vi "driveTrainControl.vi"(6 "driveTrainKillButton":bool, 7 "ClosedLoopMaxOutput":dbl, 8 "backRight":T1={"DeviceStatus"={"status"=FALSE, "code"=0, "source"=""}, "Type"=enum."PWM", "PWM"={"Digital Module"=enum."Digital Module 2", "PWM Channel"=enum."PWM 1", "DeadBand"={"Name"="", "maxPositivePwm"=0, "minPositivePwm"=0, "centerPwm"=0, "maxNegativePwm"=0, "minNegativePwm"=0, "angularRange"=0}}, "CAN"={"Device Number"=0, "Control Mode"=enum."Percent VBus", "Semaphore"=refnum, "Max Vout"=12.0}, "Invert"=FALSE, "TransformRef"=refnum, "InvTransformRef"=refnum}, 9 "backLeft":T1={"DeviceStatus"={"status"=FALSE, "code"=0, "source"=""}, "Type"=enum."PWM", "PWM"={"Digital Module"=enum."Digital Module 2", "PWM Channel"=enum."PWM 1", "DeadBand"={"Name"="", "maxPositivePwm"=0, "minPositivePwm"=0, "centerPwm"=0, "maxNegativePwm"=0, "minNegativePwm"=0, "angularRange"=0}}, "CAN"={"Device Number"=0, "Control Mode"=enum."Percent VBus", "Semaphore"=refnum, "Max Vout"=12.0}, "Invert"=FALSE, "TransformRef"=refnum, "InvTransformRef"=refnum}, 10 "frontRight":T1={"DeviceStatus"={"status"=FALSE, "code"=0, "source"=""}, "Type"=enum."PWM", "PWM"={"Digital Module"=enum."Digital Module 2", "PWM Channel"=enum."PWM 1", "DeadBand"={"Name"="", "maxPositivePwm"=0, "minPositivePwm"=0, "centerPwm"=0, "maxNegativePwm"=0, "minNegativePwm"=0, "angularRange"=0}}, "CAN"={"Device Number"=0, "Control Mode"=enum."Percent VBus", "Semaphore"=refnum, "Max Vout"=12.0}, "Invert"=FALSE, "TransformRef"=refnum, "InvTransformRef"=refnum}, 11 "frontLeft":T1={"DeviceStatus"={"status"=FALSE, "code"=0, "source"=""}, "Type"=enum."PWM", "PWM"={"Digital Module"=enum."Digital Module 2", "PWM Channel"=enum."PWM 1", "DeadBand"={"Name"="", "maxPositivePwm"=0, "minPositivePwm"=0, "centerPwm"=0, "maxNegativePwm"=0, "minNegativePwm"=0, "angularRange"=0}}, "CAN"={"Device Number"=0, "Control Mode"=enum."Percent VBus", "Semaphore"=refnum, "Max Vout"=12.0}, "Invert"=FALSE, "TransformRef"=refnum, "InvTransformRef"=refnum}) -> (0 "backRight":T1={"DeviceStatus"={"status"=FALSE, "code"=0, "source"=""}, "Type"=enum."PWM", "PWM"={"Digital Module"=enum."Digital Module 1", "PWM Channel"=enum."Invalid", "DeadBand"={"Name"="", "maxPositivePwm"=0, "minPositivePwm"=0, "centerPwm"=0, "maxNegativePwm"=0, "minNegativePwm"=0, "angularRange"=0}}, "CAN"={"Device Number"=0, "Control Mode"=enum."Percent VBus", "Semaphore"=refnum, "Max Vout"=12.0}, "Invert"=FALSE, "TransformRef"=refnum, "InvTransformRef"=refnum}, 1 "backLeft":T1={"DeviceStatus"={"status"=FALSE, "code"=0, "source"=""}, "Type"=enum."PWM", "PWM"={"Digital Module"=enum."Digital Module 1", "PWM Channel"=enum."Invalid", "DeadBand"={"Name"="", "maxPositivePwm"=0, "minPositivePwm"=0, "centerPwm"=0, "maxNegativePwm"=0, "minNegativePwm"=0, "angularRange"=0}}, "CAN"={"Device Number"=0, "Control Mode"=enum."Percent VBus", "Semaphore"=refnum, "Max Vout"=12.0}, "Invert"=FALSE, "TransformRef"=refnum, "InvTransformRef"=refnum}, 2 "frontRight":T1={"DeviceStatus"={"status"=FALSE, "code"=0, "source"=""}, "Type"=enum."PWM", "PWM"={"Digital Module"=enum."Digital Module 1", "PWM Channel"=enum."Invalid", "DeadBand"={"Name"="", "maxPositivePwm"=0, "minPositivePwm"=0, "centerPwm"=0, "maxNegativePwm"=0, "minNegativePwm"=0, "angularRange"=0}}, "CAN"={"Device Number"=0, "Control Mode"=enum."Percent VBus", "Semaphore"=refnum, "Max Vout"=12.0}, "Invert"=FALSE, "TransformRef"=refnum, "InvTransformRef"=refnum}, 3 "frontLeft":T1={"DeviceStatus"={"status"=FALSE, "code"=0, "source"=""}, "Type"=enum."PWM", "PWM"={"Digital Module"=enum."Digital Module 1", "PWM Channel"=enum."Invalid", "DeadBand"={"Name"="", "maxPositivePwm"=0, "minPositivePwm"=0, "centerPwm"=0, "maxNegativePwm"=0, "minNegativePwm"=0, "angularRange"=0}}, "CAN"={"Device Number"=0, "Control Mode"=enum."Percent VBus", "Semaphore"=refnum, "Max Vout"=12.0}, "Invert"=FALSE, "TransformRef"=refnum, "InvTransformRef"=refnum}, 5 "drivetrainMaxOutput":dbl)   [LabVIEW 2012]
uses:
  <vilib>/Rock Robotics/WPI/MotorControl/WPI_MotorControlDeviceRef.ctl
  <vilib>/Rock Robotics/SystemInterfaces/Typedef/FPGA_TypedefDigitalModule.ctl
  <vilib>/Rock Robotics/SystemInterfaces/DIO/FPGA_DIOPWMChannel.ctl
  <vilib>/Rock Robotics/WPI/PWM/WPI_PWMDeadband.ctl
  <vilib>/Rock Robotics/WPI/CAN/Jaguar/SubVIs/WPI_CANJaguar_ControlMode.ctl
  <vilib>/Rock Robotics/WPI/PWM/WPI_PWMTransform_ConPane.ctl
  <vilib>/Rock Robotics/WPI/CAN/Jaguar/SubVIs/WPI_CANJaguar_SpeedReference.ctl
  2013NewCan/Robot Global Data.vi
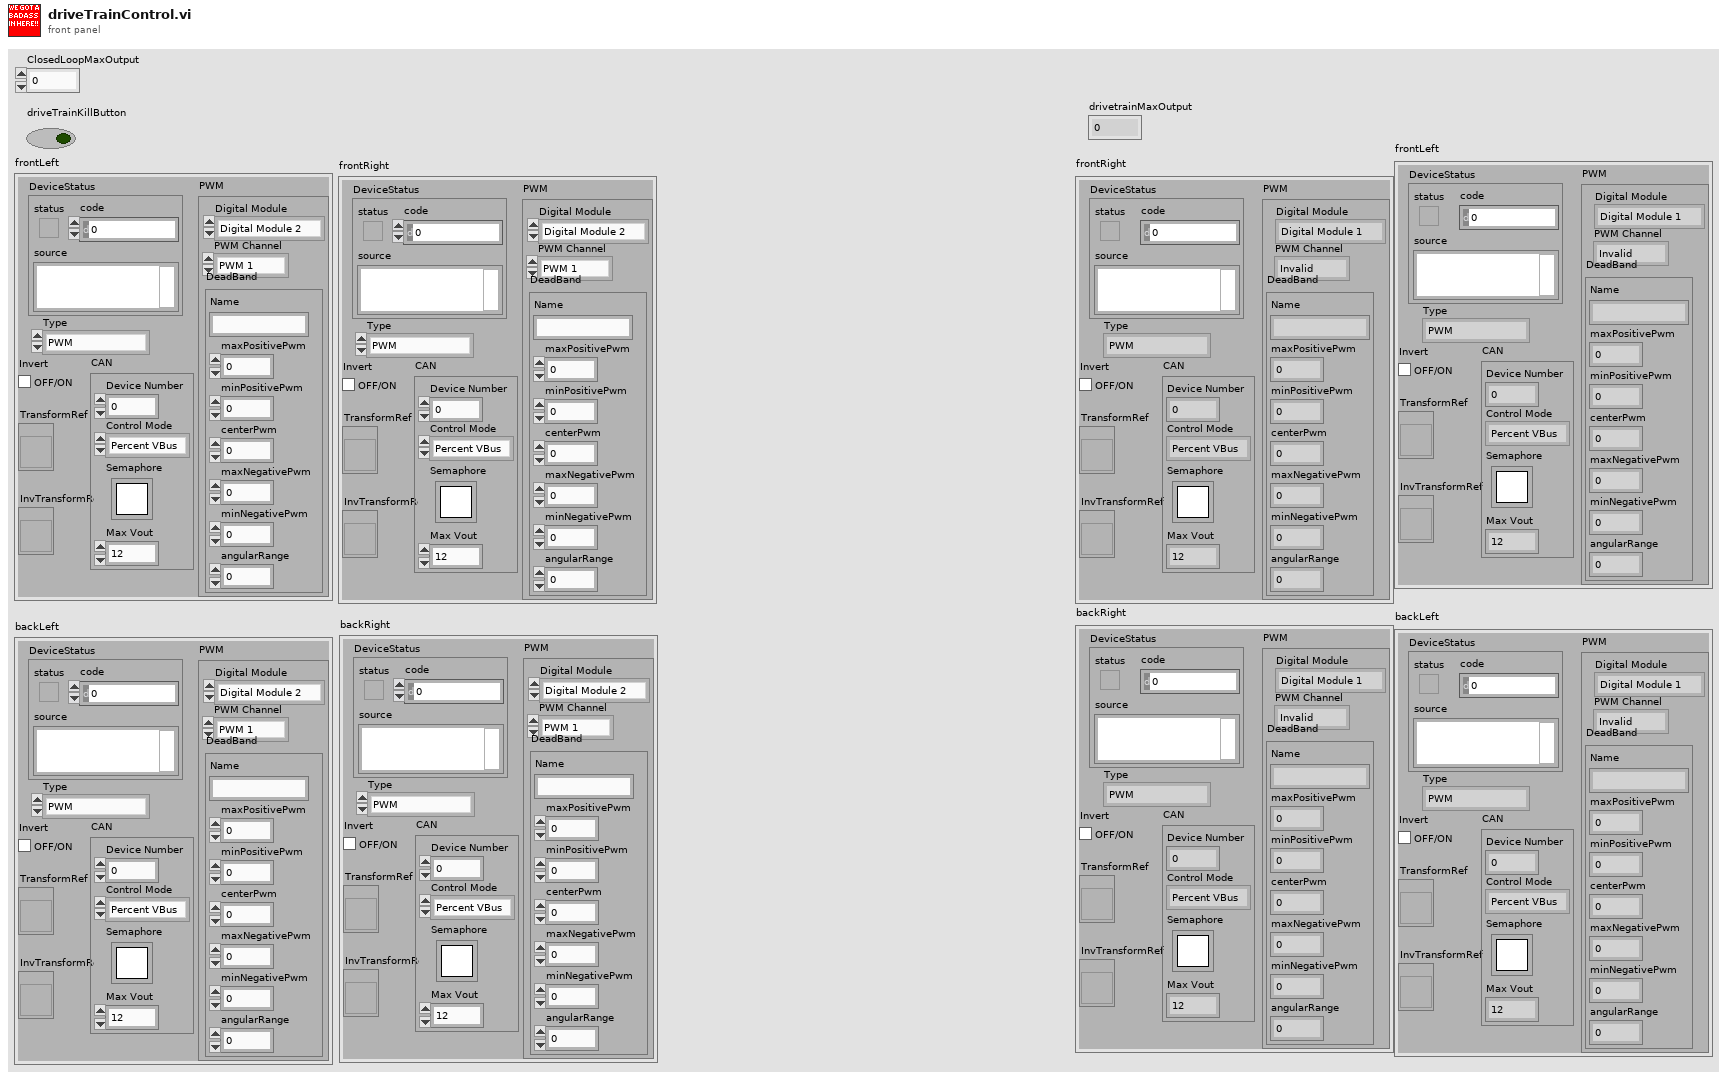
[diagram p1: front panel]
types:
  T1 = typedef "WPI_MotorControlDeviceRef.ctl" = cluster{"DeviceStatus":errorcluster, "Type":enum16{"PWM", "CAN"}, "PWM":cluster{"Digital Module":T2, "PWM Channel":T3, "DeadBand":T4}, "CAN":cluster{"Device Number":u8, "Control Mode":T5, "Semaphore":T6, "Max Vout":dbl}, "Invert":bool, "TransformRef":T7, "InvTransformRef":T7}
  T2 = typedef "FPGA_TypedefDigitalModule.ctl" = enum16{"Digital Module 1", "Digital Module 2"}
  T3 = typedef "FPGA_DIOPWMChannel.ctl" = enum8{"PWM 1", "PWM 2", "PWM 3", "PWM 4", "PWM 5", "PWM 6", "PWM 7", "PWM 8", "PWM 9", "PWM 10", "Invalid"}
  T4 = typedef "WPI_PWMDeadband.ctl" = cluster{"Name":string, "maxPositivePwm":i32, "minPositivePwm":i32, "centerPwm":i32, "maxNegativePwm":i32, "minNegativePwm":i32, "angularRange":u16}
  T5 = typedef "WPI_CANJaguar_ControlMode.ctl" = enum8{"Percent VBus", "Current", "Speed", "Position", "Voltage"}
  T6 = typedef "Semaphore RefNum" = refnum<k1>
  T7 = typedef "WPI_PWMTransform_ConPane.ctl" = refnum<vi>
  T8 = typedef "WPI_CANJaguar_SpeedReference.ctl" = u8
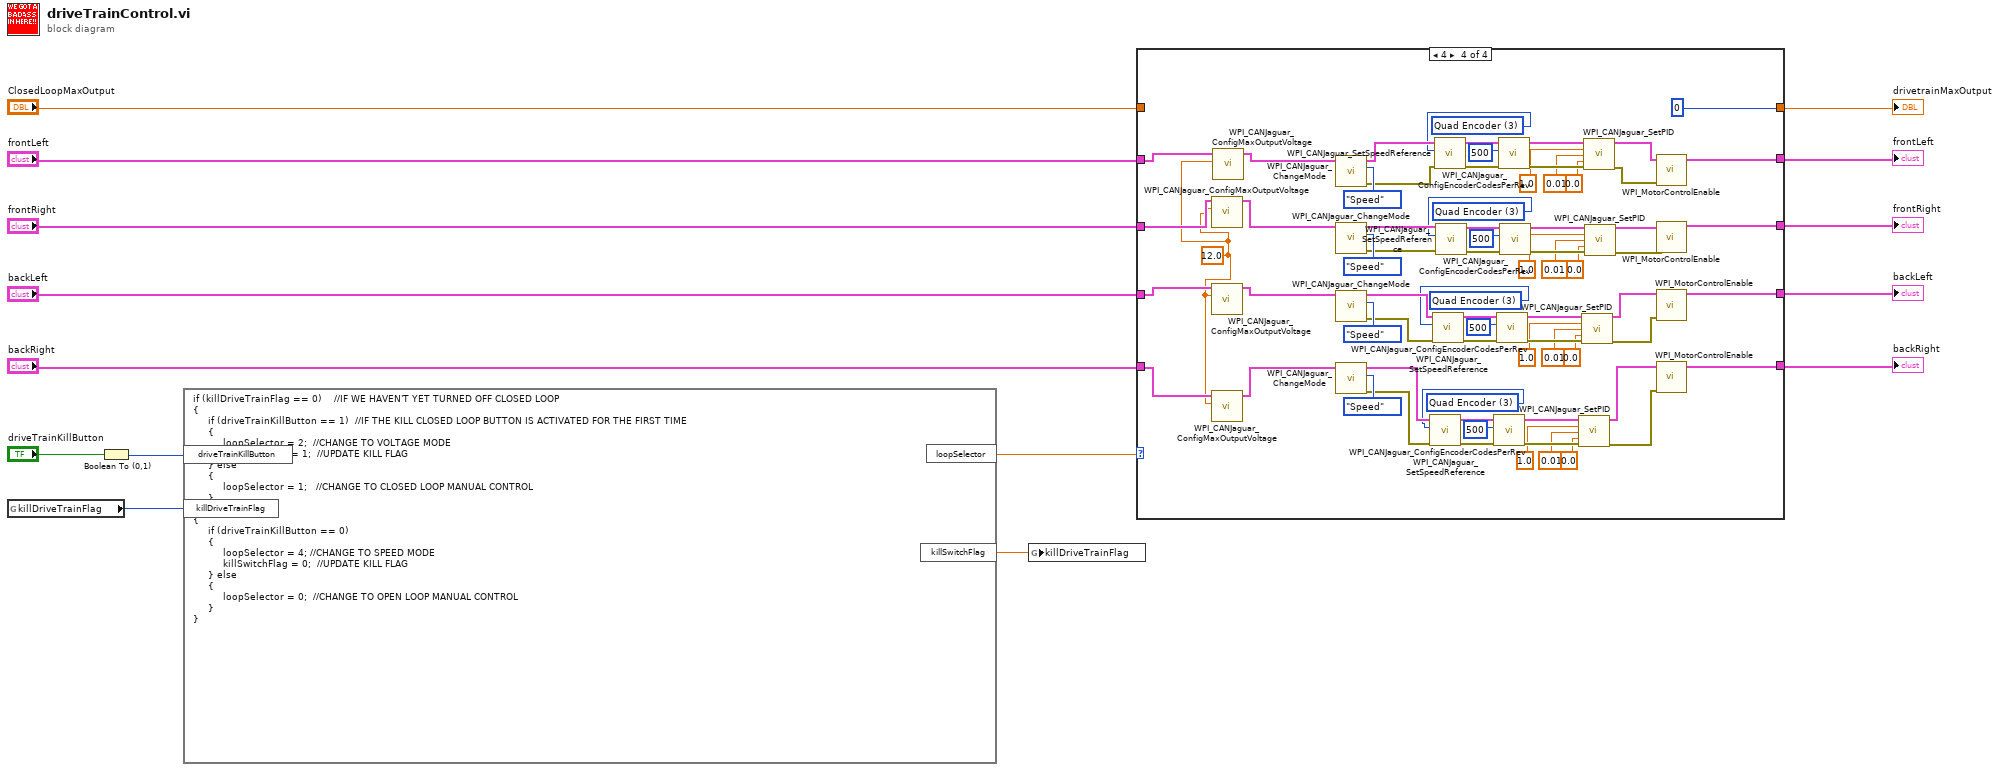
[diagram p0: block diagram]
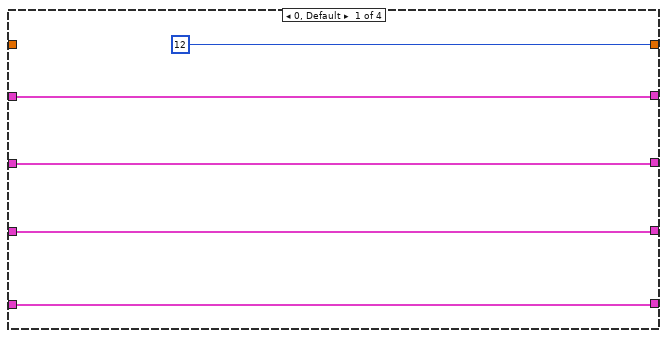
[diagram p2: hidden frame]
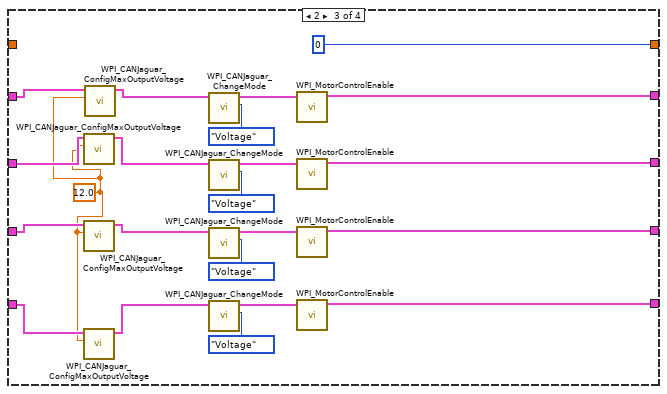
[diagram p4: hidden frame]
diagram:
  n1 = global read "Robot Global Data.vi" "killDriveTrainFlag"() -> (w9:i8)
  n2 = Boolean To (0,1)(Boolean="driveTrainKillButton") -> (0, 1=w11:i16)
  n3 = formula code="if (killDriveTrainFlag == 0)    //IF WE HAVEN'T YET TURNED OFF CLOSED LOOP\n{\n     if (driveTrainKillButton == 1)  //IF THE KILL CLOSED LOOP BUTTON IS ACTIVATED FOR THE FIRST TIME\n     {\n          loopSelector = 2;  //CHANGE TO VOLTAGE MODE\n          killSwitchFlag = 1;  //UPDATE KILL FLAG\n     } else\n     {\n          loopSelector = 1;   //CHANGE TO CLOSED LOOP MANUAL CONTROL\n     }\n} else\n{\n     if (driveTrainKillButton == 0)\n     {\n          loopSelector = 4; //CHANGE TO SPEED MODE\n          killSwitchFlag = 0;  //UPDATE KILL FLAG\n     } else\n     {\n          loopSelector = 0;  //CHANGE TO OPEN LOOP MANUAL CONTROL\n     }\n}"("driveTrainKillButton"=w11, "killDriveTrainFlag"=w9) -> ("loopSelector"=w1:dbl, "killSwitchFlag"=w8:dbl)
  n4 = global write "Robot Global Data.vi" "killDriveTrainFlag"(w8) -> ()
  n5 = case shown="4" w1 {
    tunnel: "frontLeft" -> [w20 w24 w34 w108]
    tunnel: "frontRight" -> [w19 w23 w33 w107]
    tunnel: "backLeft" -> [w18 w22 w32 w106]
    tunnel: "backRight" -> [w17 w21 w31 w105]
    tunnel: [w18 w22 w39 w113] -> w7
    tunnel: [w19 w23 w38 w112] -> w6
    tunnel: [w20 w24 w37 w111] -> w5
    tunnel: [w17 w21 w36 w110] -> w4
    tunnel: [12 w25 0 0] -> w3
    tunnel: "ClosedLoopMaxOutput" -> [_ w25 _ _]
    frame 0, Default {
    }
    frame 1 {
    }
    frame 2 {
      w26 = 12.0 ("Maximum Output Voltage")
      n6 = call <vilib>:"WPI_CANJaguar_ConfigMaxOutputVoltage.vi"("Maximum Output Voltage"=w26, "CAN Jaguar Ref"=w33) -> ("CAN Jaguar Ref Out"=w28:T1)  [unwired: 8 in, 1 out]
      n7 = call <vilib>:"WPI_CANJaguar_ConfigMaxOutputVoltage.vi"("Maximum Output Voltage"=w26, "CAN Jaguar Ref"=w32) -> ("CAN Jaguar Ref Out"=w29:T1)  [unwired: 8 in, 1 out]
      n8 = call <vilib>:"WPI_CANJaguar_ConfigMaxOutputVoltage.vi"("Maximum Output Voltage"=w26, "CAN Jaguar Ref"=w31) -> ("CAN Jaguar Ref Out"=w30:T1)  [unwired: 8 in, 1 out]
      n9 = call <vilib>:"WPI_CANJaguar_ConfigMaxOutputVoltage.vi"("Maximum Output Voltage"=w26, "CAN Jaguar Ref"=w34) -> ("CAN Jaguar Ref Out"=w27:T1)  [unwired: 8 in, 1 out]
      n10 = call <vilib>:"WPI_CANJaguar_ChangeMode.vi"("Control Mode"=WPI_CANJaguar_ControlMode."Voltage", "CAN Jaguar Ref"=w27) -> ("CAN Jaguar Ref Out"=w46:T1)  [unwired: 8 in, 1 out]
      n11 = call <vilib>:"WPI_CANJaguar_ChangeMode.vi"("Control Mode"=WPI_CANJaguar_ControlMode."Voltage", "CAN Jaguar Ref"=w28) -> ("CAN Jaguar Ref Out"=w44:T1)  [unwired: 8 in, 1 out]
      n12 = call <vilib>:"WPI_CANJaguar_ChangeMode.vi"("Control Mode"=WPI_CANJaguar_ControlMode."Voltage", "CAN Jaguar Ref"=w29) -> ("CAN Jaguar Ref Out"=w42:T1)  [unwired: 8 in, 1 out]
      n13 = call <vilib>:"WPI_CANJaguar_ChangeMode.vi"("Control Mode"=WPI_CANJaguar_ControlMode."Voltage", "CAN Jaguar Ref"=w30) -> ("CAN Jaguar Ref Out"=w40:T1)  [unwired: 8 in, 1 out]
      n14 = call <vilib>:"WPI_MotorControlEnable.vi"("CAN Jaguar Ref"=w46) -> ("CAN Jaguar Ref Out"=w37:T1)  [unwired: 9 in, 1 out]
      n15 = call <vilib>:"WPI_MotorControlEnable.vi"("CAN Jaguar Ref"=w44) -> ("CAN Jaguar Ref Out"=w38:T1)  [unwired: 9 in, 1 out]
      n16 = call <vilib>:"WPI_MotorControlEnable.vi"("CAN Jaguar Ref"=w42) -> ("CAN Jaguar Ref Out"=w39:T1)  [unwired: 9 in, 1 out]
      n17 = call <vilib>:"WPI_MotorControlEnable.vi"("CAN Jaguar Ref"=w40) -> ("CAN Jaguar Ref Out"=w36:T1)  [unwired: 9 in, 1 out]
    }
    frame 4 {
      w48 = T8 3 items=["Encoder"=0, "Inv Encoder"=2, "Quad Encoder"=3, "None"=255] ("Speed Reference")
      w49 = T8 3 items=["Encoder"=0, "Inv Encoder"=2, "Quad Encoder"=3, "None"=255] ("Speed Reference")
      w50 = T8 3 items=["Encoder"=0, "Inv Encoder"=2, "Quad Encoder"=3, "None"=255] ("Speed Reference")
      w51 = T8 3 items=["Encoder"=0, "Inv Encoder"=2, "Quad Encoder"=3, "None"=255] ("Speed Reference")
      w100 = 12.0 ("Maximum Output Voltage")
      n18 = call <vilib>:"WPI_CANJaguar_ConfigMaxOutputVoltage.vi"("Maximum Output Voltage"=w100, "CAN Jaguar Ref"=w107) -> ("CAN Jaguar Ref Out"=w102:T1)  [unwired: 8 in, 1 out]
      n19 = call <vilib>:"WPI_CANJaguar_ConfigMaxOutputVoltage.vi"("Maximum Output Voltage"=w100, "CAN Jaguar Ref"=w106) -> ("CAN Jaguar Ref Out"=w103:T1)  [unwired: 8 in, 1 out]
      n20 = call <vilib>:"WPI_CANJaguar_ConfigMaxOutputVoltage.vi"("Maximum Output Voltage"=w100, "CAN Jaguar Ref"=w105) -> ("CAN Jaguar Ref Out"=w104:T1)  [unwired: 8 in, 1 out]
      n21 = call <vilib>:"WPI_CANJaguar_ConfigMaxOutputVoltage.vi"("Maximum Output Voltage"=w100, "CAN Jaguar Ref"=w108) -> ("CAN Jaguar Ref Out"=w101:T1)  [unwired: 8 in, 1 out]
      n22 = call <vilib>:"WPI_CANJaguar_ChangeMode.vi"("Control Mode"=WPI_CANJaguar_ControlMode."Speed", "CAN Jaguar Ref"=w101) -> ("error out"=w65:errorcluster, "CAN Jaguar Ref Out"=w67:T1)  [unwired: 8 in]
      n23 = call <vilib>:"WPI_CANJaguar_ChangeMode.vi"("Control Mode"=WPI_CANJaguar_ControlMode."Speed", "CAN Jaguar Ref"=w102) -> ("error out"=w64:errorcluster, "CAN Jaguar Ref Out"=w66:T1)  [unwired: 8 in]
      n24 = call <vilib>:"WPI_CANJaguar_ChangeMode.vi"("Control Mode"=WPI_CANJaguar_ControlMode."Speed", "CAN Jaguar Ref"=w103) -> ("error out"=w62:errorcluster, "CAN Jaguar Ref Out"=w63:T1)  [unwired: 8 in]
      n25 = call <vilib>:"WPI_CANJaguar_ChangeMode.vi"("Control Mode"=WPI_CANJaguar_ControlMode."Speed", "CAN Jaguar Ref"=w104) -> ("error out"=w60:errorcluster, "CAN Jaguar Ref Out"=w61:T1)  [unwired: 8 in]
      n26 = call <vilib>:"WPI_CANJaguar_SetSpeedReference.vi"("error in (no error)"=w60, "Speed Reference"=w48, "CAN Jaguar Ref"=w61) -> ("error out"=w70:errorcluster, "CAN Jaguar Ref Out"=w69:T1)  [unwired: 7 in]
      n27 = call <vilib>:"WPI_CANJaguar_SetSpeedReference.vi"("error in (no error)"=w62, "Speed Reference"=w49, "CAN Jaguar Ref"=w63) -> ("error out"=w78:errorcluster, "CAN Jaguar Ref Out"=w77:T1)  [unwired: 7 in]
      n28 = call <vilib>:"WPI_CANJaguar_SetSpeedReference.vi"("error in (no error)"=w65, "Speed Reference"=w51, "CAN Jaguar Ref"=w67) -> ("error out"=w94:errorcluster, "CAN Jaguar Ref Out"=w93:T1)  [unwired: 7 in]
      n29 = call <vilib>:"WPI_CANJaguar_SetSpeedReference.vi"("error in (no error)"=w64, "Speed Reference"=w50, "CAN Jaguar Ref"=w66) -> ("error out"=w86:errorcluster, "CAN Jaguar Ref Out"=w85:T1)  [unwired: 7 in]
      n30 = call <vilib>:"WPI_CANJaguar_ConfigEncoderCodesPerRev.vi"("error in (no error)"=w70, "Encoder Codes Per Rev"=u16 500, "CAN Jaguar Ref"=w69) -> ("error out"=w74:errorcluster, "CAN Jaguar Ref Out"=w68:T1)  [unwired: 7 in]
      n31 = call <vilib>:"WPI_CANJaguar_ConfigEncoderCodesPerRev.vi"("error in (no error)"=w78, "Encoder Codes Per Rev"=u16 500, "CAN Jaguar Ref"=w77) -> ("error out"=w82:errorcluster, "CAN Jaguar Ref Out"=w76:T1)  [unwired: 7 in]
      n32 = call <vilib>:"WPI_CANJaguar_ConfigEncoderCodesPerRev.vi"("error in (no error)"=w94, "Encoder Codes Per Rev"=u16 500, "CAN Jaguar Ref"=w93) -> ("error out"=w98:errorcluster, "CAN Jaguar Ref Out"=w92:T1)  [unwired: 7 in]
      n33 = call <vilib>:"WPI_CANJaguar_ConfigEncoderCodesPerRev.vi"("error in (no error)"=w86, "Encoder Codes Per Rev"=u16 500, "CAN Jaguar Ref"=w85) -> ("error out"=w90:errorcluster, "CAN Jaguar Ref Out"=w84:T1)  [unwired: 7 in]
      n34 = call <vilib>:"WPI_CANJaguar_SetPID.vi"("CAN Jaguar Ref"=w68, "P"=1.0, "I"=0.01, "D"=0.0, "error in (no error)"=w74) -> ("CAN Jaguar Ref Out"=w53:T1, "error out"=w52:errorcluster)  [unwired: 9 in]
      n35 = call <vilib>:"WPI_CANJaguar_SetPID.vi"("CAN Jaguar Ref"=w76, "P"=1.0, "I"=0.01, "D"=0.0, "error in (no error)"=w82) -> ("CAN Jaguar Ref Out"=w55:T1, "error out"=w54:errorcluster)  [unwired: 9 in]
      n36 = call <vilib>:"WPI_CANJaguar_SetPID.vi"("CAN Jaguar Ref"=w92, "P"=1.0, "I"=0.01, "D"=0.0, "error in (no error)"=w98) -> ("CAN Jaguar Ref Out"=w56:T1, "error out"=w57:errorcluster)  [unwired: 9 in]
      n37 = call <vilib>:"WPI_CANJaguar_SetPID.vi"("CAN Jaguar Ref"=w84, "P"=1.0, "I"=0.01, "D"=0.0, "error in (no error)"=w90) -> ("CAN Jaguar Ref Out"=w59:T1, "error out"=w58:errorcluster)  [unwired: 9 in]
      n38 = call <vilib>:"WPI_MotorControlEnable.vi"("error in (no error)"=w57, "CAN Jaguar Ref"=w56) -> ("CAN Jaguar Ref Out"=w111:T1)  [unwired: 8 in, 1 out]
      n39 = call <vilib>:"WPI_MotorControlEnable.vi"("error in (no error)"=w58, "CAN Jaguar Ref"=w59) -> ("CAN Jaguar Ref Out"=w112:T1)  [unwired: 8 in, 1 out]
      n40 = call <vilib>:"WPI_MotorControlEnable.vi"("error in (no error)"=w54, "CAN Jaguar Ref"=w55) -> ("CAN Jaguar Ref Out"=w113:T1)  [unwired: 8 in, 1 out]
      n41 = call <vilib>:"WPI_MotorControlEnable.vi"("error in (no error)"=w52, "CAN Jaguar Ref"=w53) -> ("CAN Jaguar Ref Out"=w110:T1)  [unwired: 8 in, 1 out]
    }
  }
  "frontLeft" <- w5
  "frontRight" <- w6
  "backLeft" <- w7
  "backRight" <- w4
  "drivetrainMaxOutput" <- w3
